vi "Pcre2SubstringFromSubjectByName8 (ba).vi"(8 "error in":errorcluster, 9 "Name":string, 10 "Subject":string, 11 "pMatchData":u64 format="%.0x") -> (0 "error out":errorcluster, 3 "pMatchData":u64 format="%.0x", 4 "AfterSubstring":string, 5 "BeforeSubstring":string)   [LabVIEW 2021, in "libpcre2-8.lvlib"]
uses:
  libpcre2-8.lvlib
  Pcre2ErrorNull.vi
  Pcre2FnkCallError.vi
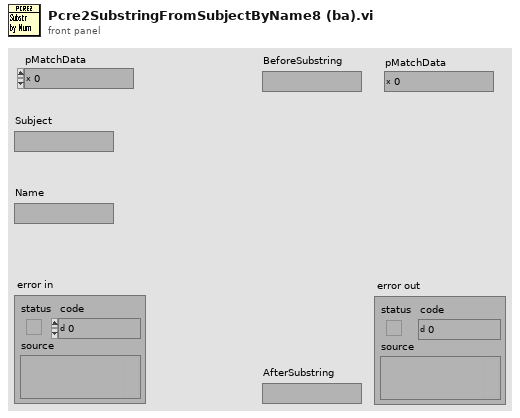
[diagram p1: front panel]
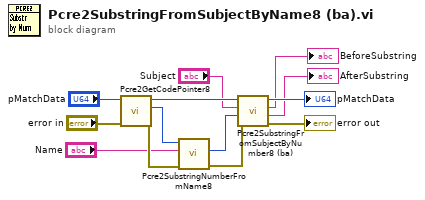
[diagram p0: block diagram]
diagram:
  n1 = call "Pcre2GetCodePointer8.vi"("error in"="error in", "pMatchData"="pMatchData") -> ("error out"=w12:errorcluster, "pCode"=w13:u64, "pMatchData"=w8:u64)  [unwired: 7 in]
  n2 = call "Pcre2SubstringNumberFromName8.vi"("error in"=w12, "Name"="Name", "pCode"=w13) -> ("error out"=w6:errorcluster, "Number"=w5:i32)  [unwired: 6 in, 1 out]
  n3 = call "Pcre2SubstringFromSubjectByNumber8 (ba).vi"("error in"=w6, "Number"=w5, "Subject"="Subject", "pMatchData"=w8) -> ("error out"=→"error out":errorcluster, "AfterSubstring"=→"AfterSubstring":string, "BeforeSubstring"=→"BeforeSubstring":string, "pMatchData"=→"pMatchData":u64)  [unwired: 4 in]
